vi "题目7.vi"() -> ()   [LabVIEW 2017]
uses:
  <vilib>/Utility/file.llb/Write Delimited Spreadsheet (DBL).vi
panel:
  out "波形图":dynamicdata(graph)
  out "数组":dbl[](array[numeric])
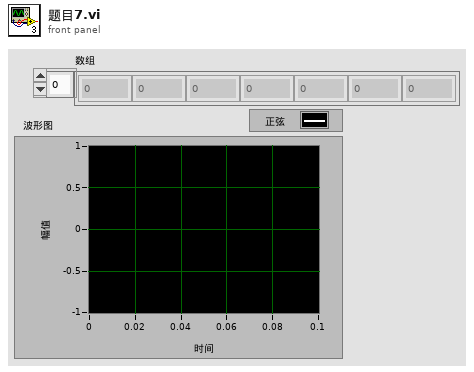
[diagram p1: front panel]
types:
  T1 = enum16{"open", "replace", "create", "open or create", "replace or create", "replace or create with confirmation"}
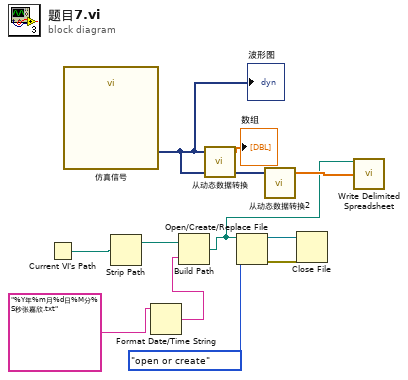
[diagram p0: block diagram]
diagram:
  n1 = Current VI's Path() -> (path=w9:path)
  n2 = call "仿真信号"() -> ("正弦"=w1:dynamicdata)  [unwired: 14 in, 1 out]
  "波形图" <- w1
  n3 = Strip Path(path=w9) -> (stripped path=w10:path)  [unwired: 1 out]
  n4 = Format Date/Time String(time format string (%c)="%Y年%m月%d日%M分%S秒张嘉欣.txt" ("名称或相对路径")) -> (date/time string=w3:string)  [unwired: 2 in]
  n5 = Build Path(base path=w10, name or relative path=w3) -> (appended path=w4:path)
  n6 = call "从动态数据转换"("Dynamic Data Type"=w1) -> ("Array"=→"数组":dbl[])  [unwired: 3 in]
  n7 = Open/Create/Replace File(file path (use dialog)=w4, operation (0:open)=T1."open or create" ("操作(0:open)")) -> (refnum out=w6:refnum<file>, error out=w7:errorcluster)  [unwired: 4 in, 1 out]
  n8 = call "从动态数据转换2"("Dynamic Data Type"=w1) -> ("Array"=w5:dbl[])  [unwired: 3 in]
  n9 = Close File(refnum=w6, error in=w7) -> ()  [unwired: 2 out]
  n10 = call-poly <vilib>:"Write Delimited Spreadsheet.vi"("file path (dialog if empty)"=w4, "1D data"=w5) -> ()  [unwired: 12 in, 2 out]
